vi "PostStep Chamber Steptype.vi"(10 "Chamber data in":T1, 11 "Sequence Context In":refnum<k7>) -> (0 "error out":errorcluster, 2 "Chamber data out":T1, 3 "Report Text":string)   [LabVIEW 2023, in "LTT_TeststandSteptypes.lvlib"]
uses:
  LTT_TeststandSteptypes.lvlib
  Control/Chamber Step Status.ctl
  Control/Chamber Step Option.ctl
  GlobalVariable/GlobalVariableData.vi
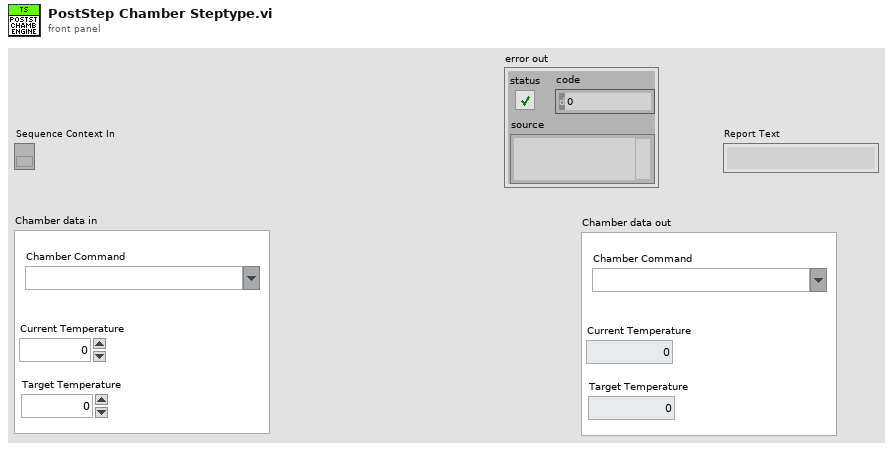
[diagram p1: front panel]
types:
  T1 = typedef "LTT_TeststandSteptypes.lvlib/Chamber Step Status.ctl" = cluster{"Current Temperature":dbl, "Target Temperature":dbl, "Chamber Command":T2}
  T2 = typedef "LTT_TeststandSteptypes.lvlib/Chamber Step Option.ctl" = string
  T3 = cluster{"Chamber Present Temp":dbl, "Chamber Target Temp":dbl, "Chamber RTD Temp":dbl}
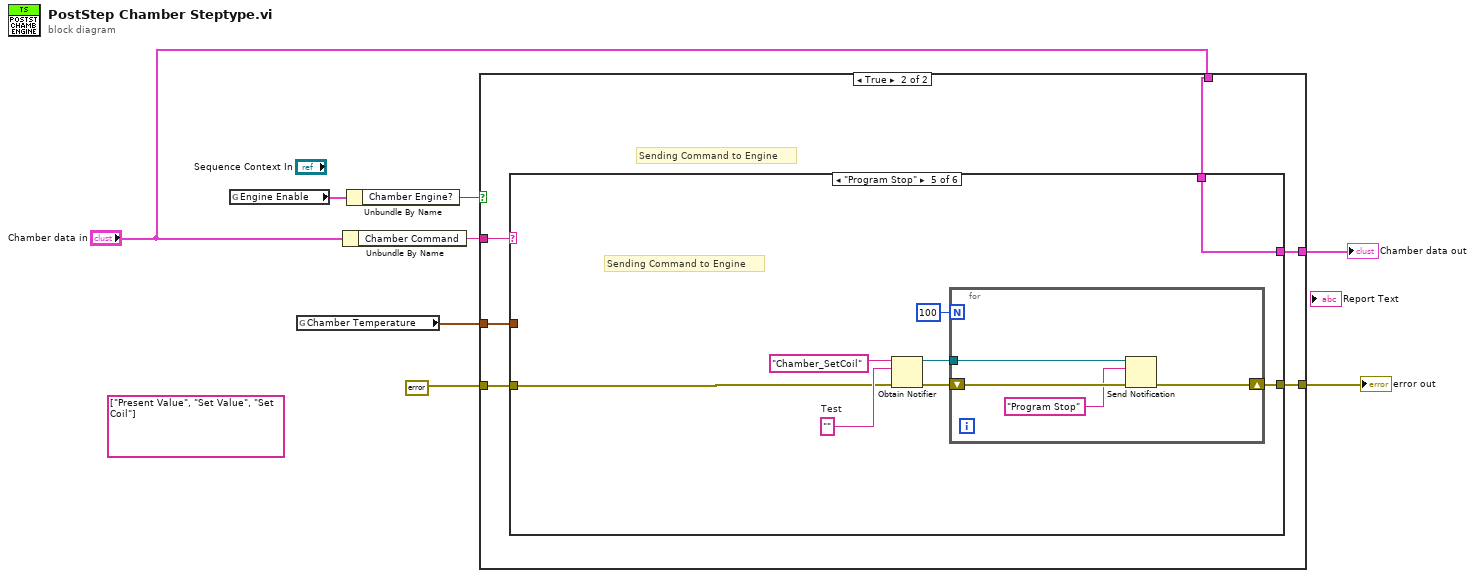
[diagram p0: block diagram]
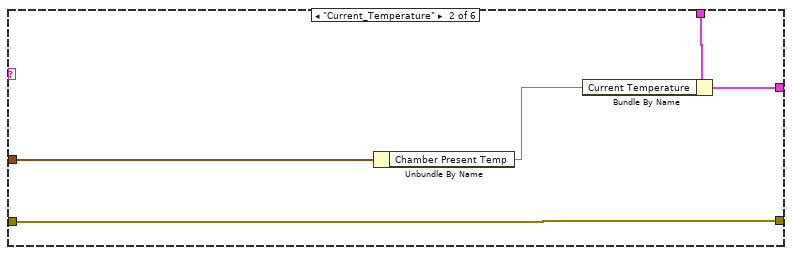
[diagram p4: hidden frame]
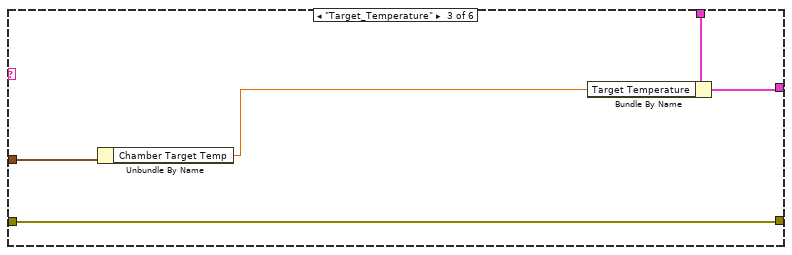
[diagram p5: hidden frame]
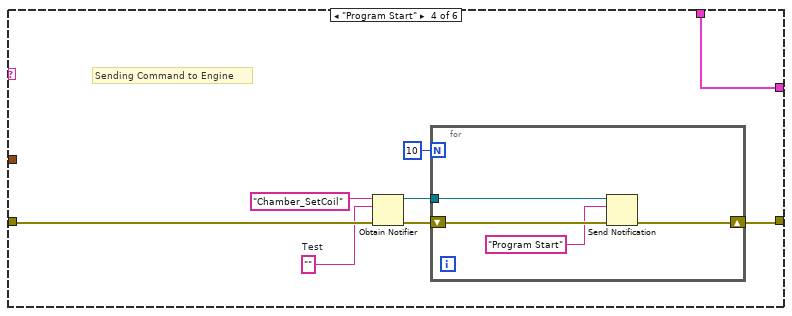
[diagram p6: hidden frame]
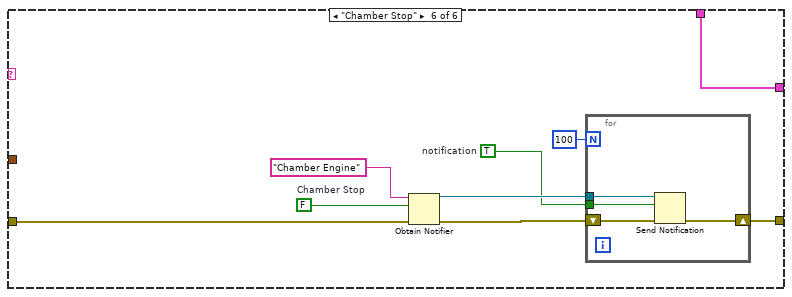
[diagram p7: hidden frame]
diagram:
  (unwired) string[] ["Present Value", "Set Value", "Set Coil"]
  n1 = global read "GlobalVariableData.vi" "Engine Enable"() -> (w4:cluster{"Chamber Engine?":bool})
  n2 = global read "GlobalVariableData.vi" "Chamber Temperature"() -> (w3:T3)
  n3 = Unbundle By Name("Chamber data in") -> ("Chamber Command"=w6:T2)
  n4 = Unbundle By Name(w4) -> ("Chamber Engine?"=w2:bool)
  n5 = case shown="True" w2 {
    tunnel: errorcluster {"status"=FALSE, "code"=0, "source"=""} ("error in (no error)") -> [w9 w16]
    tunnel: [w9 w15] -> w7
    tunnel: w6 -> [_ w14]
    tunnel: [w10 w13] -> w5
    tunnel: w3 -> [_ w12]
    tunnel: "Chamber data in" -> [w10 w11]
    frame False {
    }
    frame True {
      # "Sending Command to Engine"
      n6 = case shown="\"Program Stop\"" w14 {
        tunnel: w16 -> [w18 w20 w28 w36 w44 w59]
        tunnel: [w18 w20 w28 w31 w43 w55] -> w15
        tunnel: w11 -> [w17 w23 w26 w30 w42 w53]
        tunnel: [w17 w22 w27 w30 w42 w53] -> w13
        tunnel: w12 -> [_ w19 w25 _ _ _]
        frame "", Default {
        }
        frame "Current_Temperature" {
          n7 = Unbundle By Name(w19) -> ("Chamber Present Temp"=w21:dbl)
          n8 = Bundle By Name(cluster=w23, "Current Temperature"=w21) -> (w22:T1)
        }
        frame "Target_Temperature" {
          n9 = Unbundle By Name(w25) -> ("Chamber Target Temp"=w24:dbl)
          n10 = Bundle By Name(cluster=w26, "Target Temperature"=w24) -> (w27:T1)
        }
        frame "Program Start" {
          w34 = ""  # Test
          # "Sending Command to Engine"
          n11 = Obtain Notifier(name (unnamed)="Chamber_SetCoil", notification data type=w34, error in (no error)=w36) -> (notifier out=w33:refnum<notifier>, error out=w32:errorcluster)  [unwired: 1 in, 1 out]
          n12 = for {
            N: 10 -> [_]
            tunnel: w33 -> [w40]
            shift-right: [w38] -> w31
            shift-left: w32 -> [w39]
            n13 = Send Notification(notification="Program Start", notifier=w40, error in (no error)=w39) -> (error out=w38:errorcluster)  [unwired: 1 out]
          }
        }
        frame "Program Stop" {
          w47 = ""  # Test
          # "Sending Command to Engine"
          n14 = Obtain Notifier(name (unnamed)="Chamber_SetCoil", notification data type=w47, error in (no error)=w44) -> (notifier out=w46:refnum<notifier>, error out=w45:errorcluster)  [unwired: 1 in, 1 out]
          n15 = for {
            N: 100 -> [_]
            tunnel: w46 -> [w52]
            shift-right: [w50] -> w43
            shift-left: w45 -> [w51]
            n16 = Send Notification(notification="Program Stop", notifier=w52, error in (no error)=w51) -> (error out=w50:errorcluster)  [unwired: 1 out]
          }
        }
        frame "Chamber Stop" {
          w56 = TRUE  # notification
          w60 = FALSE  # Chamber Stop
          n17 = Obtain Notifier(name (unnamed)="Chamber Engine", notification data type=w60, error in (no error)=w59) -> (notifier out=w58:refnum<notifier>, error out=w57:errorcluster)  [unwired: 1 in, 1 out]
          n18 = for {
            N: 100 -> [_]
            tunnel: w58 -> [w65]
            tunnel: w56 -> [w63]
            shift-right: [w62] -> w55
            shift-left: w57 -> [w64]
            n19 = Send Notification(notification=w63, notifier=w65, error in (no error)=w64) -> (error out=w62:errorcluster)  [unwired: 1 out]
          }
        }
      }
    }
  }
  "error out" <- w7
  "Chamber data out" <- w5
